vi "GUI_CH1_Comm_TCPIP.vi"() -> ()   [LabVIEW 2018]
uses:
  RxTx/RxTx.lvclass
  TCPIP/TCPIP.lvclass
panel:
  in  "Channel:":u16=1
  in  "stop":bool
  out "error out 4":errorcluster
  out "error out 2":errorcluster
  out "error out":errorcluster
  in  "RxTx.lvclass 2":refnum<class "RxTx.lvclass">
  in  "remote port":u16=59041
  in  "IP":string="200.131.64.49"
  in  "TCPIP.lvclass":refnum<class "TCPIP.lvclass">
  in  "RxTx.lvclass":refnum<class "RxTx.lvclass">
  # "GEI - Channel 1 communication"
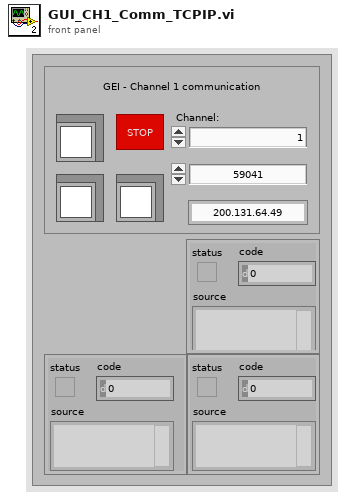
[diagram p1: front panel]
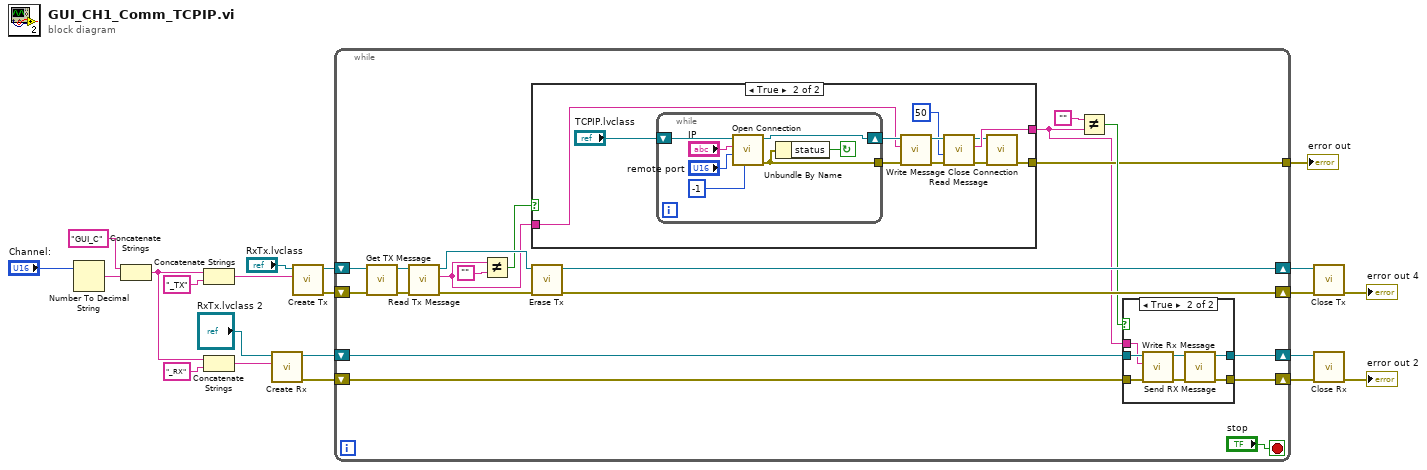
[diagram p0: block diagram]
diagram:
  n1 = Number To Decimal String(number="Channel:") -> (decimal integer string=w8:string)  [unwired: 1 in]
  n2 = Concatenate Strings("GUI_C", w8) -> (w2:string)
  n3 = Concatenate Strings(w2, "_TX" ("Reader Name")) -> (w1:string)
  n4 = Concatenate Strings(w2, "_RX" ("Reader Name")) -> (w5:string)
  n5 = call "Create Rx.vi"("Reader Name"=w5, "RxTx in"="RxTx.lvclass 2") -> ("error out"=w15:errorcluster, "RxTx out"=w14:refnum<class "RxTx.lvclass">)  [unwired: 8 in]
  n6 = call "Create Tx.vi"("Writer Name"=w1, "RxTx in"="RxTx.lvclass") -> ("error out"=w20:errorcluster, "RxTx out"=w21:refnum<class "RxTx.lvclass">)  [unwired: 8 in]
  n7 = while {
    shift-right: [w33] -> w18
    shift-left: w20 -> [w38]
    shift-right: [w35] -> w19
    shift-left: w21 -> [w39]
    shift-right: [w28] -> w13
    shift-left: w14 -> [w29]
    shift-right: [w27] -> w12
    shift-left: w15 -> [w30]
    tunnel: [w24] -> w11
    stop <- "stop" stop-if-true
    n8 = call "Get TX Message.vi"("error in (no error)"=w38, "RxTx in"=w39) -> ("error out"=w41:errorcluster, "RxTx out"=w40:refnum<class "RxTx.lvclass">)  [unwired: 8 in]
    n9 = call "Read Tx Message.vi"("error in (no error)"=w41, "RxTx in"=w40) -> ("error out"=w34:errorcluster, "Tx Message"=w32:string, "RxTx out"=w36:refnum<class "RxTx.lvclass">)  [unwired: 7 in]
    n10 = Not Equal?(x=w32, y="") -> (x != y?=w31:bool)
    n11 = case shown="True" w31 {
      tunnel: w32 -> [_ w60]
      tunnel: [_ w52] -> w24
      tunnel: [_ w58] -> w23
      frame False {
      }
      frame True {
        n12 = while {
          shift-right: [w67] -> w61
          shift-left: "TCPIP.lvclass" -> [w68]
          tunnel: [w62] -> w51
          stop <- w65 continue-if-true
          n13 = call "Open Connection.vi"("timeout"=-1, "remote port"="remote port", "IP"="IP", "TCPIP in"=w68) -> ("error out"=w62:errorcluster, "TCPIP out"=w67:refnum<class "TCPIP.lvclass">)  [unwired: 6 in]
          n14 = Unbundle By Name(w62) -> ("status"=w65:bool)
        }
        n15 = call "Write Message.vi"("error in (no error)"=w51, "Message"=w60, "TCPIP in"=w61) -> ("error out"=w56:errorcluster, "TCPIP out"=w57:refnum<class "TCPIP.lvclass">)  [unwired: 7 in]
        n16 = call "Read Message.vi"("error in (no error)"=w56, "timeout"=50, "TCPIP in"=w57) -> ("error out"=w59:errorcluster, "Message"=w58:string, "TCPIP out"=w54:refnum<class "TCPIP.lvclass">)  [unwired: 6 in]
        n17 = call "Close Connection.vi"("error in (no error)"=w59, "TCPIP in"=w54) -> ("error out"=w52:errorcluster)  [unwired: 8 in, 1 out]
      }
    }
    n18 = call "Erase Tx.vi"("error in (no error)"=w34, "RxTx in"=w36) -> ("error out"=w33:errorcluster, "RxTx out"=w35:refnum<class "RxTx.lvclass">)  [unwired: 8 in]
    n19 = Not Equal?(x="", y=w23) -> (x != y?=w25:bool)
    n20 = case shown="True" w25 {
      tunnel: w30 -> [w42 w48]
      tunnel: w29 -> [w43 w47]
      tunnel: [w43 w46] -> w28
      tunnel: [w42 w45] -> w27
      tunnel: w23 -> [_ w44]
      frame False {
      }
      frame True {
        n21 = call "Write Rx Message.vi"("error in (no error)"=w48, "Rx Message"=w44, "RxTx in"=w47) -> ("error out"=w50:errorcluster, "RxTx out"=w49:refnum<class "RxTx.lvclass">)  [unwired: 7 in]
        n22 = call "Send RX Message.vi"("error in (no error)"=w50, "RxTx in"=w49) -> ("error out"=w45:errorcluster, "RxTx out"=w46:refnum<class "RxTx.lvclass">)  [unwired: 8 in]
      }
    }
  }
  "error out" <- w11
  n23 = call "Close Tx.vi"("error in (no error)"=w18, "RxTx in"=w19) -> ("error out"=→"error out 4":errorcluster)  [unwired: 8 in, 1 out]
  n24 = call "Close Rx.vi"("error in (no error)"=w12, "RxTx in"=w13) -> ("error out"=→"error out 2":errorcluster)  [unwired: 8 in, 1 out]
